vi "KB-laser 计算同心度.vi"(10 "小圆圆心":T1 {"Average SNR (dB)" format="%.2f"; "Average Strength" format="%.2f"; "Roundness (Real-World)" format="%.2f"; "Radius (Real-World)" format="%.2f"; "Center (Real-World)"."Y" format="%.2f"; "Center (Real-World)"."X" format="%.2f"; "Radius (Pixels)" format="%.2f"; "Center (Pixels)"."Y" format="%.2f"; "Center (Pixels)"."X" format="%.2f"}, 11 "大圆圆心":T1 {"Average SNR (dB)" format="%.2f"; "Average Strength" format="%.2f"; "Roundness (Real-World)" format="%.2f"; "Radius (Real-World)" format="%.2f"; "Center (Real-World)"."Y" format="%.2f"; "Center (Real-World)"."X" format="%.2f"; "Radius (Pixels)" format="%.2f"; "Center (Pixels)"."Y" format="%.2f"; "Center (Pixels)"."X" format="%.2f"}) -> (3 "sqrt(x)":sgl)   [LabVIEW 2015]
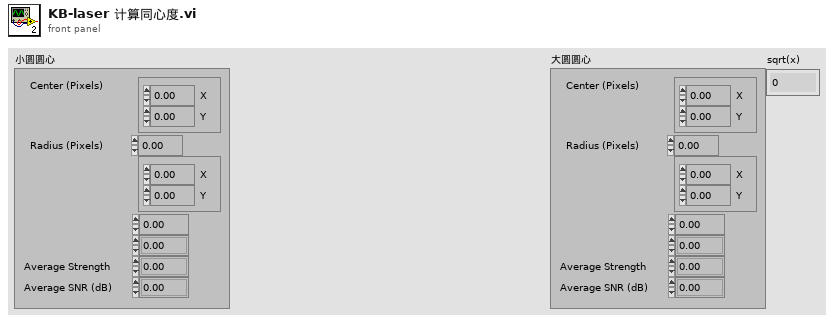
[diagram p1: front panel]
types:
  T1 = cluster{"Center (Pixels)":cluster{"X":sgl, "Y":sgl}, "Radius (Pixels)":dbl, "Center (Real-World)":cluster{"X":sgl, "Y":sgl}, "Radius (Real-World)":dbl, "Roundness (Real-World)":dbl, "Average Strength":dbl, "Average SNR (dB)":dbl}
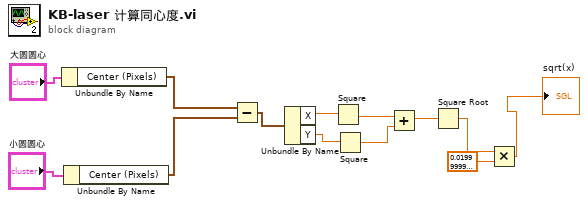
[diagram p0: block diagram]
diagram:
  n1 = Unbundle By Name("大圆圆心") -> ("Center (Pixels)"=w5:cluster{"X":sgl, "Y":sgl})
  n2 = Unbundle By Name("小圆圆心") -> ("Center (Pixels)"=w4:cluster{"X":sgl, "Y":sgl})
  n3 = Subtract(x=w5, y=w4) -> (x-y=w11:cluster{"X":sgl, "Y":sgl})
  n4 = Unbundle By Name(w11) -> ("X"=w10:sgl, "Y"=w9:sgl)
  n5 = Square(x=w10) -> (x^2=w8:sgl)
  n6 = Square(x=w9) -> (x^2=w7:sgl)
  n7 = Add(x=w8, y=w7) -> (x+y=w6:sgl)
  n8 = Square Root(x=w6) -> (sqrt(x)=w2:sgl)
  n9 = Multiply(x=w2, y=sgl 0.02) -> (x*y=→"sqrt(x)":sgl)
